vi "Convert Controls to Arrays.vi"(10 "Ctl Properties":T1[](array[typedef])) -> (1 "Indicator Array":string[][](array[string]), 3 "Control Array":string[][](array[string]))   [LabVIEW 2023, in "VI Properties Editor.lvlib"]
uses:
  VI Properties Editor.lvlib
  CTLs/Control Properties.ctl
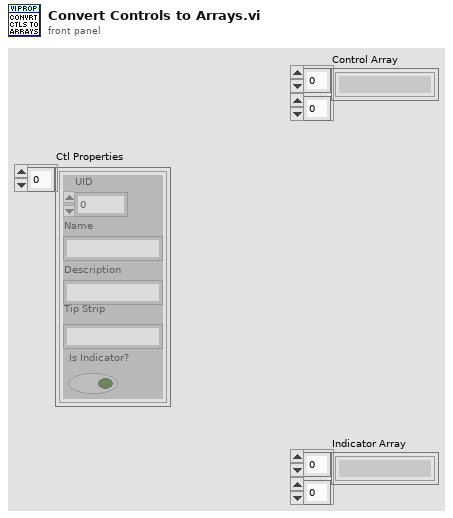
[diagram p1: front panel]
types:
  T1 = typedef "VI Properties Editor.lvlib/Control Properties.ctl" = cluster{"UID":i32, "Name":string, "Description":string, "Tip Strip":string, "Is Indicator?":bool}
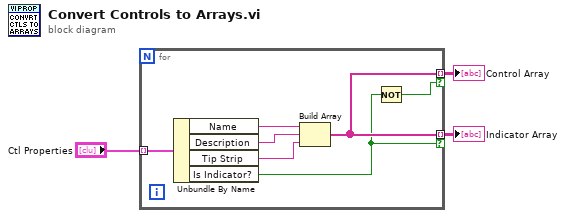
[diagram p0: block diagram]
diagram:
  n1 = for {
    tunnel: [w10] -> w2 mode=indexing if=w4
    tunnel: [w10] -> w1 mode=indexing if=w5
    tunnel: "Ctl Properties" -> [w9] mode=indexing
    n2 = Unbundle By Name(w9) -> ("Name"=w8:string, "Description"=w7:string, "Tip Strip"=w6:string, "Is Indicator?"=w5:bool)
    n3 = Build Array(w8, w7, w6) -> (w10:string[])
    n4 = Not(x=w5) -> (.not. x?=w4:bool)
  }
  "Control Array" <- w2
  "Indicator Array" <- w1
